vi "PCO_GetFrameRate.vi"(8 "error in (no error)":errorcluster {"code" format="%x"}, 11 "ph":u64) -> (0 "error out":errorcluster {"code" format="%x"}, 1 "wFrameRateStatus":u16, 2 "ErrorMessage":i32 format="%x", 3 "ph out":u64, 4 "dwFrameRateExposure":u32, 5 "dwFrameRate":u32)   [LabVIEW 2019, in "SDK.lvlib" / "TimingControl.lvlib"]
doc: "<b>Description:</b>\nThis function returns the current frame rate and exposure time settings of the camera.\nReturned values are only valid if last timing command was PCO_SetFrameRate.\n\n<b>Supported camera type:</b>\npco.edge, pco.dimax\n\n<b>Descriptor dependency:</b>\ndwGeneralCapsDESC1: SETFRAMERATE_ENABLED"
uses:
  TimingControl.lvlib
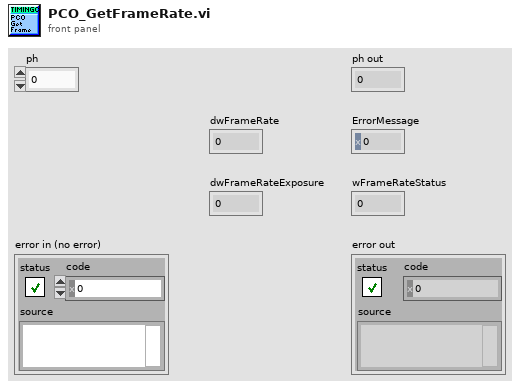
[diagram p1: front panel]
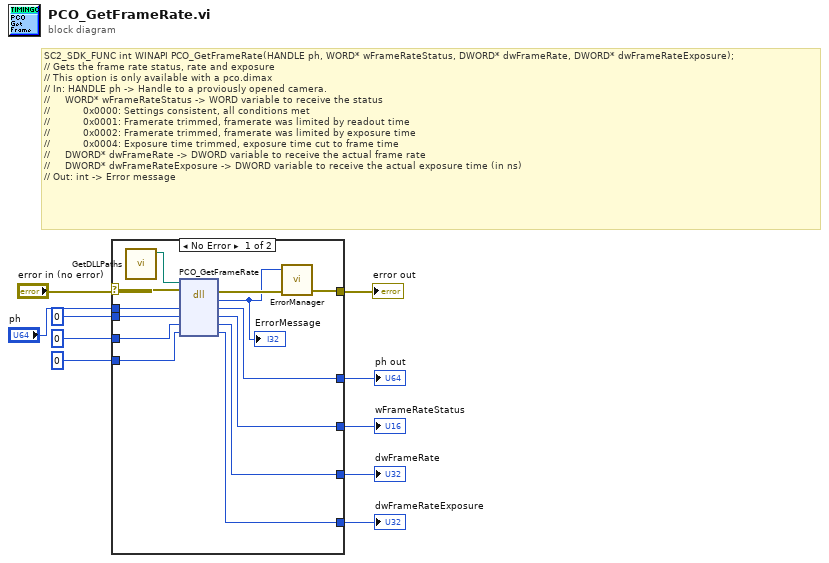
[diagram p0: block diagram]
diagram:
  # "SC2_SDK_FUNC int WINAPI PCO_GetFrameRate(HANDLE ph, WORD* wFrameRateStatus, DWORD* dwFrameRate, DWORD* dwFrameRateExposure);\n// Gets the frame rate status, rate and exposure\n// This option is only available with a pco.dimax\n// In: HANDLE ph -> Handle to a proviously opened camera.\n//     WORD* wFrameRateStatus -> WORD variable to receive the status\n//           0x0000: Settings consistent, all conditions met\n//           0x0001: Framerate trimmed, framerate was limited by readout time\n//           0x0002: Framerate trimmed, framerate was limited by exposure time\n//           0x0004: Exposure time trimmed, exposure time cut to frame time\n//     DWORD* dwFrameRate -> DWORD variable to receive the actual frame rate\n//     DWORD* dwFrameRateExposure -> DWORD variable to receive the actual exposure time (in ns)\n// Out: int -> Error message"
  n1 = case shown="No Error" "error in (no error)" {
    selector: "error in (no error)" -> [w15 w28]
    tunnel: "ph" -> [w23 w27]
    tunnel: [w22 w27] -> w9
    tunnel: u16 0 ("wFrameRateStatus") -> [w21 w26]
    tunnel: [w20 w26] -> w7
    tunnel: u32 0 ("dwFrameRate") -> [w19 w25]
    tunnel: [w18 w25] -> w5
    tunnel: u32 0 ("dwFrameRateExposure") -> [w17 w24]
    tunnel: [w16 w24] -> w3
    tunnel: [w13 w28] -> w2
    frame No Error {
      n2 = call "GetDLLPaths.vi"() -> ("SC2_Cam_Path"=w11:path)  [unwired: 8 in, 3 out]
      n3 = dll-call lib="?" fn="PCO_GetFrameRate"(path in=w11, error in=w15, "ph"=w23, "wFrameRateStatus"=w21, "dwFrameRate"=w19, "dwFrameRateExposure"=w17) -> (error out=w14:errorcluster, "return type"=w12:i32, "ph"=w22:u64, "wFrameRateStatus"=w20:u16, "dwFrameRate"=w18:u32, "dwFrameRateExposure"=w16:u32)  [unwired: 1 in, 1 out]
      "ErrorMessage" <- w12
      n4 = call "ErrorManager.vi"("error in (no error)"=w14, "error code"=w12) -> ("error out"=w13:errorcluster)  [unwired: 2 in, 1 out]
    }
    frame Error {
    }
  }
  "ph out" <- w9
  "wFrameRateStatus" <- w7
  "dwFrameRate" <- w5
  "dwFrameRateExposure" <- w3
  "error out" <- w2
